vi "Gui_About.vi"(8 "error in (no error)":errorcluster) -> (0 "error out":errorcluster)   [LabVIEW 2020]
doc: "This VI displays the version of the current application.\nThis VI runs both in development mode and run-time mode, and calls the fileVersionInfo.llb"
uses:
  <vilib>/Platform/fileVersionInfo.llb/FileVersionInformation.ctl
panel:
  in  "OK":bool
  out "FileVersionInfo Out":T1
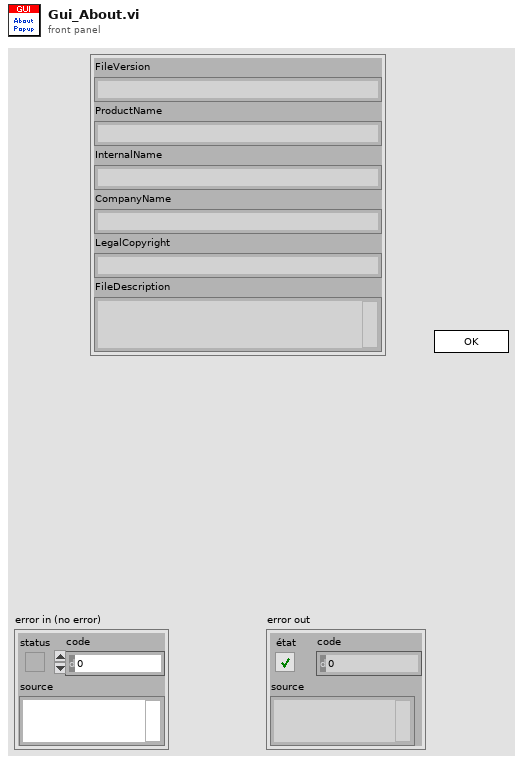
[diagram p1: front panel]
types:
  T1 = typedef "FileVersionInformation.ctl" = cluster{"FileVersion":string, "ProductName":string, "InternalName":string, "CompanyName":string, "LegalCopyright":string, "FileDescription":string}
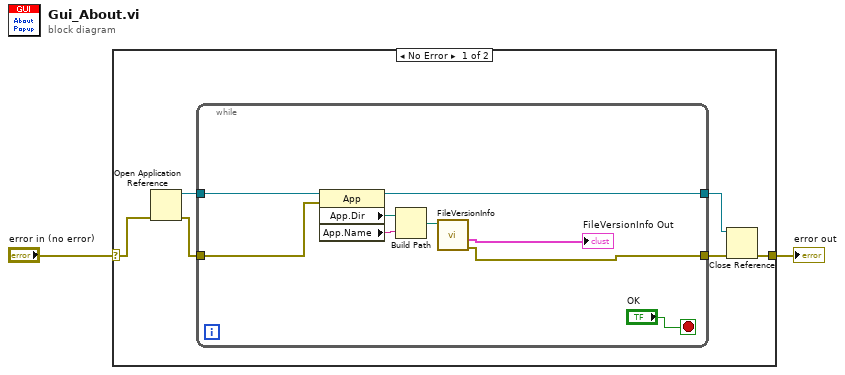
[diagram p0: block diagram]
diagram:
  n1 = case shown="No Error" "error in (no error)" {
    selector: "error in (no error)" -> [w4 w18]
    tunnel: [w5 w18] -> w1
    frame No Error {
      n2 = Open Application Reference(8:w4) -> (0:w3:errorcluster, 3:w8:refnum<vi>)  [unwired: 3 in]
      n3 = while {
        tunnel: w3 -> [w15]
        tunnel: [w14] -> w6
        tunnel: w8 -> [w17]
        tunnel: [w16] -> w7
        stop <- "OK" stop-if-true
        n4 = property class="App"(reference=w17, error in=w15) -> (reference out=w16:refnum<vi>, "App.Dir"=w13:path, "App.Name"=w12:string)  [unwired: 1 out]
        n5 = Build Path(base path=w13, name or relative path=w12) -> (appended path=w11:path)
        n6 = call <vilib>:"FileVersionInfo.vi"("Application Path in"=w11) -> ("error out"=w14:errorcluster, "FileVersionInfo Out"=→"FileVersionInfo Out":T1)  [unwired: 7 in, 2 out]
      }
      n7 = Close Reference(reference=w7, error in (no error)=w6) -> (error out=w5:errorcluster)
    }
    frame Error {
    }
  }
  "error out" <- w1
